vi "Handle Exception.vi"(7 "Processing In":refnum<class "Processing.lvclass">, 8 "error in (no error)":errorcluster, 11 "BadRequestException in":refnum<class "BadRequestException.lvclass">) -> (0 "error out":errorcluster, 5 "Processing":refnum<class "Processing.lvclass">)   [LabVIEW 2020, in "HTTP Server.lvlib" / "BadRequestException.lvclass"]
uses:
  BadRequestException.lvclass
  Processing/Processing.lvclass
  BadRequestException.lvclass/BadRequestException.ctl
  <vilib>/Utility/error.llb/DialogType.ctl
  <vilib>/IlluminatedG/IG HTTP Utils/HTTP Utils/Response/Response.lvclass
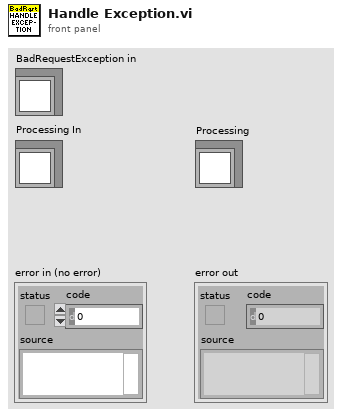
[diagram p1: front panel]
types:
  T1 = typedef "DialogType.ctl" = u16
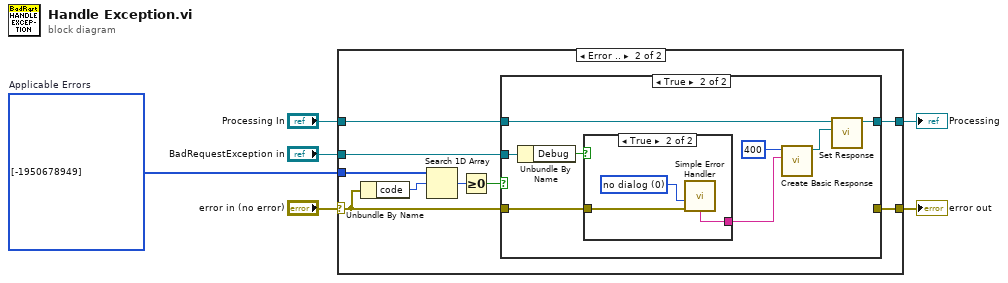
[diagram p0: block diagram]
diagram:
  w5 = i32[] [-1950678949]  # Applicable Errors
  n1 = case shown="Error .." "error in (no error)" {
    selector: "error in (no error)" -> [w8 w14]
    tunnel: w5 -> [_ w17]
    tunnel: "BadRequestException in" -> [_ w12]
    tunnel: [w8 w11] -> w3
    tunnel: [w7 w10] -> w2
    tunnel: "Processing In" -> [w7 w9]
    frame No Error {
    }
    frame Error {
      n2 = Unbundle By Name(w14) -> ("code"=w16:i32)
      n3 = Search 1D Array(1D array=w17, element=w16) -> (index of element=w15:i32)  [unwired: 1 in]
      n4 = Greater Or Equal To 0?(x=w15) -> (x >= 0?=w13:bool)
      n5 = case shown="True" w13 {
        tunnel: w14 -> [w19 w25]
        tunnel: w12 -> [_ w27]
        tunnel: [w19 _] -> w11
        tunnel: [w18 w20] -> w10
        tunnel: w9 -> [w18 w22]
        frame False {
        }
        frame True {
          n6 = Unbundle By Name(w27) -> ("Debug"=w26:bool)
          n7 = case shown="True" w26 {
            tunnel: w25 -> [_ w30]
            tunnel: [_ w28] -> w23
            frame False {
            }
            frame True {
              w29 = T1 0 items=["no dialog", "OK message", "continue or stop message", "OK message + warnings", "continue/stop + warnings"] ("type of dialog (OK msg:1)")
              n8 = call <vilib>:"Simple Error Handler.vi"("type of dialog (OK msg:1)"=w29, "error in (no error)"=w30) -> ("message"=w28:string)  [unwired: 3 in, 4 out]
            }
          }
          n9 = call <vilib>:"Create Basic Response.vi"("Payload"=w23, "Status Code"=u16 400) -> ("Response out"=w21:refnum<class "Response.lvclass">)  [unwired: 8 in, 1 out]
          n10 = call "Set Response.vi"("Response"=w21, "Processing in"=w22) -> ("Processing out"=w20:refnum<class "Processing.lvclass">)  [unwired: 9 in]
        }
      }
    }
  }
  "error out" <- w3
  "Processing" <- w2
